vi "SOFandEOF.vi"(8 "error in (no error)":errorcluster, 11 "ISO 14443 B DOWN in":refnum<class "ISO 14443 B DOWN.lvclass">) -> (0 "error out":errorcluster, 3 "ISO 14443 B DOWN out":refnum<class "ISO 14443 B DOWN.lvclass">, 5 "frame":u8[](array[numeric]))   [LabVIEW 2019, in "ISO 14443 B DOWN.lvclass"]
uses:
  ISO 14443 B DOWN.lvclass
  TypeDef/Store.ctl
  ISO 14443 B DOWN.lvclass/ISO 14443 B DOWN.ctl
  RFID system.lvclass
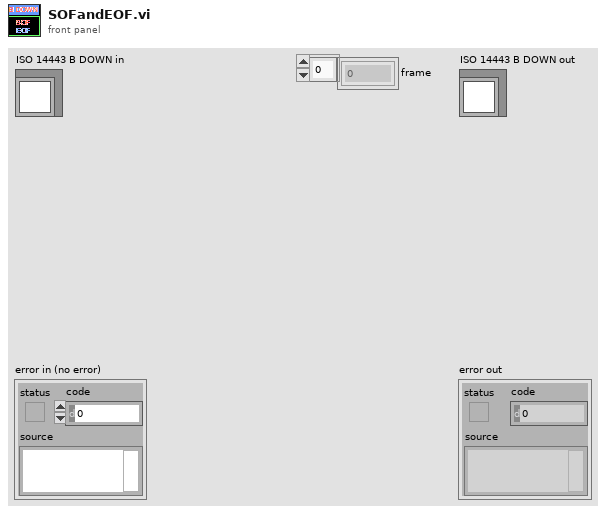
[diagram p1: front panel]
types:
  T1 = typedef "Store.ctl" = enum16{"envelope", "noise", "demSubCar", "CH_frame", "Decode", "demodulate", "in", "out", "sum", "subCarrier", "frame", "command", "encode", "modulate", "encode_UP", "modulate_up", "demod_up", "envelop_up", "sum_up", "out_up", "in_up"}
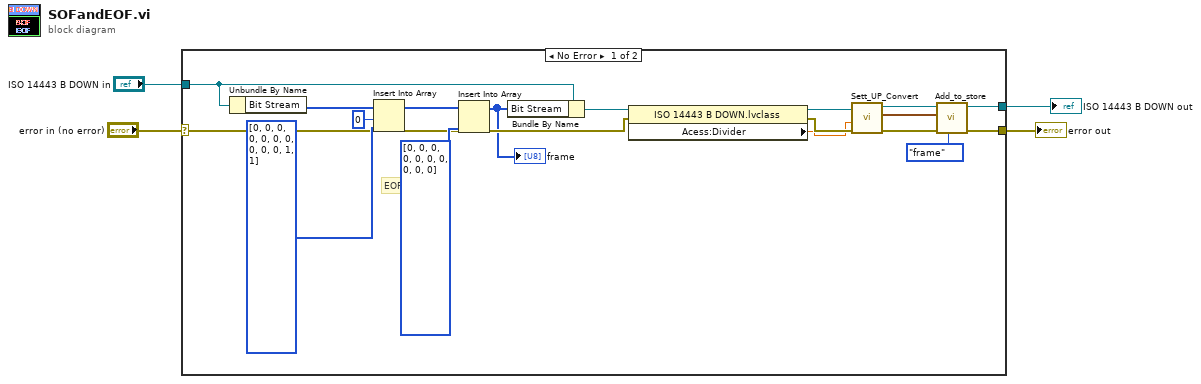
[diagram p0: block diagram]
diagram:
  n1 = case shown="No Error" "error in (no error)" {
    selector: "error in (no error)" -> [w8 w23]
    tunnel: [w12 w23] -> w3
    tunnel: "ISO 14443 B DOWN in" -> [w17 w24]
    tunnel: [w14 w24] -> w1
    frame No Error {
      # "EOF"
      # "SOF"
      n2 = Unbundle By Name(w17) -> ("Bit Stream"=w18:u8[])
      n3 = Insert Into Array(array=w18, index=0, new element=u8[] [0, 0, 0, 0, 0, 0, 0, 0, 0, 0, 1, 1] ("Bit stream out (NRZ encode)")) -> (w20:u8[])
      n4 = Insert Into Array(array=w20, new element=u8[] [0, 0, 0, 0, 0, 0, 0, 0, 0, 0] ("Bit stream out (NRZ encode)")) -> (w5:u8[])  [unwired: 1 in]
      "frame" <- w5
      n5 = Bundle By Name(cluster=w17, "Bit Stream"=w5) -> (w16:refnum<class "ISO 14443 B DOWN.lvclass">)
      n6 = property class="ISO 14443 B DOWN.lvclass"(reference=w16, error in=w8) -> (reference out=w9:refnum<class "ISO 14443 B DOWN.lvclass">, error out=w7:errorcluster, "Acess:Divider"=w6:dbl)
      n7 = call-dynamic "Sett_UP_Convert.vi"("error in (no error)"=w7, "Divider(1)"=w6, "ISO 14443 B DOWN in"=w9) -> ("error out"=w13:errorcluster, "Waveform"=w11:waveform(dbl), "ISO 14443 B DOWN out"=w15:refnum<class "ISO 14443 B DOWN.lvclass">)  [unwired: 6 in]
      n8 = call "Add_to_store.vi"("Store"=Store."frame", "error in (no error)"=w13, "Waveform"=w11, "RFID system in"=w15) -> ("error out"=w12:errorcluster, "RFID system out"=w14:refnum<class "ISO 14443 B DOWN.lvclass">)  [unwired: 6 in]
    }
    frame Error {
    }
  }
  "error out" <- w3
  "ISO 14443 B DOWN out" <- w1
